vi "WriteDataSubVi.vi"(5 "error in (no error)":errorcluster, 6 "write buffer":string, 7 "VISA resource name":refnum<visa-resource-name>) -> (0 "read buffer":string, 1 "error out":errorcluster, 2 "return count":u32, 3 "VISA resource name out":refnum<visa-resource-name>)   [LabVIEW 2024]
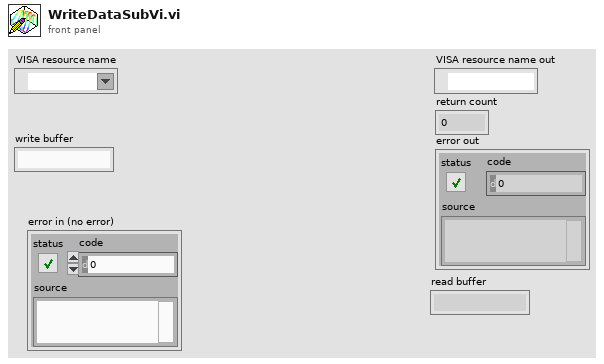
[diagram p1: front panel]
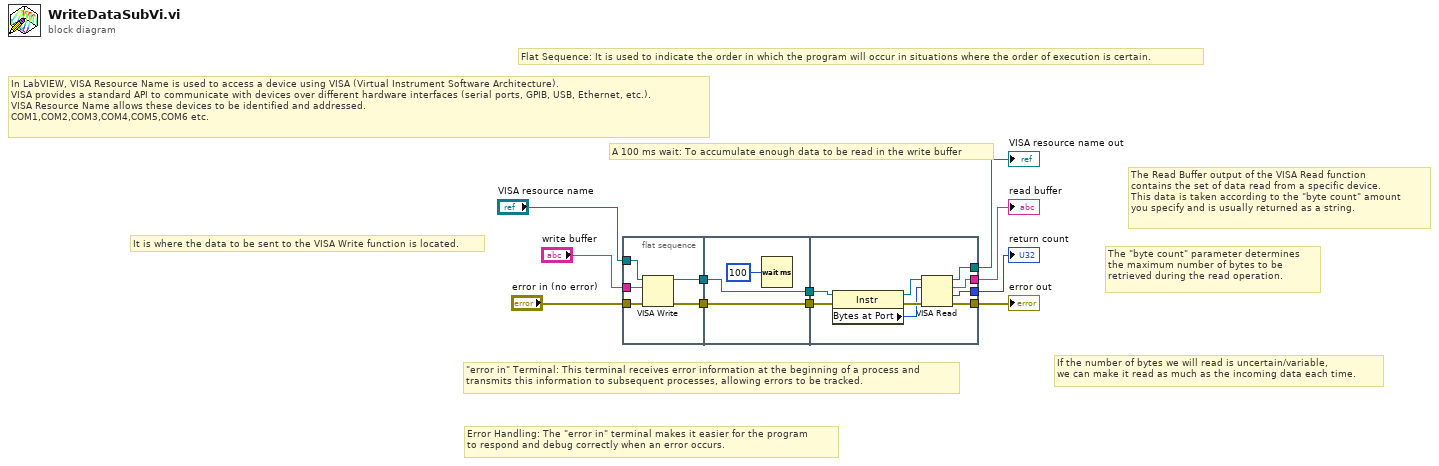
[diagram p0: block diagram]
diagram:
  # "The Read Buffer output of the VISA Read function \ncontains the set of data read from a specific device. \nThis data is taken according to the \"byte count\" amount \nyou specify and is usually returned as a string."
  # "Flat Sequence: It is used to indicate the order in which the program will occur in situations where the order of execution is certain."
  # "If the number of bytes we will read is uncertain/variable, \nwe can make it read as much as the incoming data each time."
  # "The \"byte count\" parameter determines \nthe maximum number of bytes to be \nretrieved during the read operation."
  # "In LabVIEW, VISA Resource Name is used to access a device using VISA (Virtual Instrument Software Architecture). \nVISA provides a standard API to communicate with devices over different hardware interfaces (serial ports, GPIB, USB, Ethernet, etc.). \nVISA Resource Name allows these devices to be identified and addressed.\nCOM1,COM2,COM3,COM4,COM5,COM6 etc."
  # "Error Handling: The \"error in\" terminal makes it easier for the program \nto respond and debug correctly when an error occurs."
  # "\"error in\" Terminal: This terminal receives error information at the beginning of a process and \ntransmits this information to subsequent processes, allowing errors to be tracked."
  # "A 100 ms wait: To accumulate enough data to be read in the write buffer"
  # "It is where the data to be sent to the VISA Write function is located."
  n1 = flat-sequence {
    tunnel: [w16] -> w10
    tunnel: [w15] -> w8
    tunnel: "VISA resource name" -> [w14]
    tunnel: "write buffer" -> [w13]
    tunnel: "error in (no error)" -> [w12]
    tunnel: [w18] -> w11
    tunnel: w10 -> [w18]
    tunnel: [w17] -> w9
    tunnel: w8 -> [w17]
    tunnel: w11 -> [w26]
    tunnel: w9 -> [w28]
    tunnel: [w23] -> w7
    tunnel: [w22] -> w6
    tunnel: [w21] -> w5
    tunnel: [w20] -> w4
    frame #0 {
      n2 = VISA Write(VISA resource name=w14, write buffer=w13, error in (no error)=w12) -> (VISA resource name out=w16:refnum<visa-resource-name>, error out=w15:errorcluster)  [unwired: 1 out]
    }
    frame #1 {
      n3 = Wait (ms)(milliseconds to wait=u32 100) -> ()  [unwired: 1 out]
    }
    frame #2 {
      n4 = property class="Instr"(reference=w26, error in=w28) -> (reference out=w25:refnum<visa-resource-name>, error out=w27:errorcluster, "Bytes at Port"=w24:u32)
      n5 = VISA Read(VISA resource name=w25, byte count=w24, error in (no error)=w27) -> (VISA resource name out=w23:refnum<visa-resource-name>, read buffer=w22:string, return count=w21:u32, error out=w20:errorcluster)
    }
  }
  "VISA resource name out" <- w7
  "read buffer" <- w6
  "return count" <- w5
  "error out" <- w4
